vi "Get Size of Data from TD - 3D Array (DBL) - Returns Correct Size.vi"() -> ()   [LabVIEW 2017, in "Composition.Tests.lvlib"]
uses:
  Composition.Tests.lvlib
  <vilib>/addons/_JKI Toolkits/Caraya/classes/Assert/Assert Equal Value_Variant.vi
  Composition/Composition.lvlib
  <vilib>/addons/_JKI Toolkits/Caraya/classes/Assert/Assert.lvclass
  <vilib>/addons/_JKI Toolkits/Caraya/classes/Test/Test.lvclass
panel:
  out "error out":errorcluster
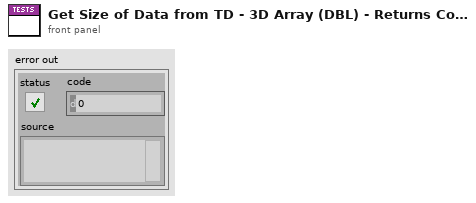
[diagram p1: front panel]
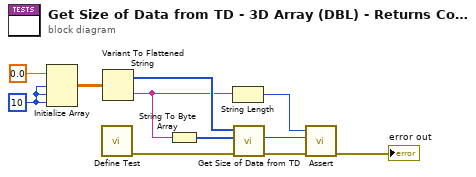
[diagram p0: block diagram]
diagram:
  w1 = 10 ("dimension size")
  n1 = Initialize Array(0.0 ("element"), w1, w1, w1) -> (w3:dbl[][][])
  n2 = call <vilib>:"Define Test.vi"() -> ("error out"=w4:errorcluster)  [unwired: 11 in]
  n3 = Variant To Flattened String(Variant=w3) -> (data string=w8:string, 1:w11:i16[])
  n4 = String To Byte Array(string=w8) -> (unsigned byte array=w10:u8[])
  n5 = String Length(string=w8) -> (length=w5:i32)
  n6 = call "Get Size of Data from TD.vi"("error in (no error)"=w4, "Data String"=w10, "Type Descriptor"=w11) -> ("error out"=w9:errorcluster, "Size of Data"=w6:i32)  [unwired: 7 in]
  n7 = call-poly <vilib>:"Assert.vi"("error in (no error)"=w9, "Y"=w6, "X"=w5) -> ("error out"=→"error out":errorcluster)  [unwired: 8 in]
